vi "Initialize Image [Body Index].vi"(8 "Error In":errorcluster, 10 "Image Name":string="Body Index Frame") -> (0 "Error Out":errorcluster, 3 "Body Index Image":T1)   [LabVIEW 2011, in "KinectOne.lvlib"]
uses:
  KinectOne.lvlib
  <vilib>/vision/Image Controls.llb/IMAQ Image.ctl
  Frame Description FGV [Body Index].vi
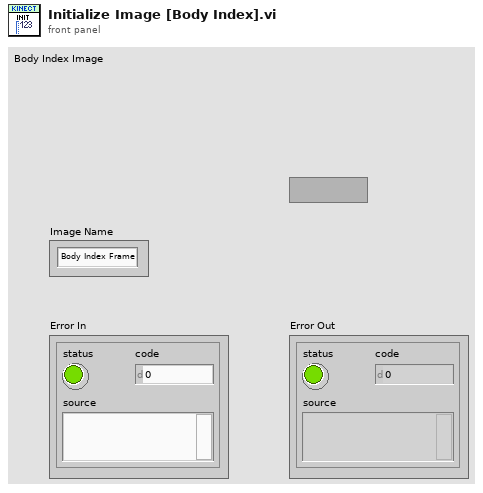
[diagram p1: front panel]
types:
  T1 = typedef "IMAQ Image.ctl" = refnum<image>
  T2 = typedef "Image Type" = u32
  T3 = typedef "KinectOne.lvlib/FrameDescription.ctl" = cluster{"BytesPerPixel":u32, "DiagonalFieldOfView":sgl, "Height":i32, "HorizontalFieldOfView":sgl, "LengthInPixels":u32, "VerticalFieldOfView":sgl, "Width":i32}
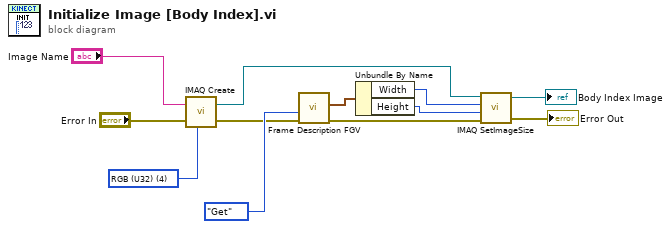
[diagram p0: block diagram]
diagram:
  w12 = T2 4 items=["Grayscale (U8)", "Grayscale (I16)", "Grayscale (SGL)", "Complex (CSG)", "RGB (U32)", "HSL (U32)", "RGB (U64)", "Grayscale (U16)"] ("Image Type")
  n1 = call "IMAQ Create"("Image Name"="Image Name", "Image Type"=w12, "error in (no error)"="Error In") -> ("New Image"=w4:T1, "error out"=w8:errorcluster)  [unwired: 2 in]
  n2 = call-poly "Frame Description FGV.vi"("error in (no error)"=w8, "Command"=enum16{"Get", "Set"}."Get") -> ("error out"=w7:errorcluster, "FrameDescription"=w9:T3)  [unwired: 8 in]
  n3 = Unbundle By Name(w9) -> ("Width"=w5:i32, "Height"=w6:i32)
  n4 = call "IMAQ SetImageSize"("error in (no error)"=w7, "Y Resolution"=w6, "X Resolution"=w5, "Image"=w4) -> ("error out"=→"Error Out":errorcluster, "Image Out"=→"Body Index Image":T1)  [unwired: 1 in]
